vi "False_Predictions.vi"(8 "error in (no error)":errorcluster, 9 "Annotations_for_ClassIdx":T4[](array[typedef]) {"Image Annotations"."BBox"."x" format="%#_4p"; "Image Annotations"."BBox"."y" format="%#_4p"; "Image Annotations"."BBox"."w" format="%#_4p"; "Image Annotations"."BBox"."h" format="%#_4p"}, 10 "TP_IOU_thresh":sgl=0.3, 11 "Detections_for_ClassIdx(by_Image)":T1[](array[typedef]) {"Image Detections"."BBox"."x" format="%#_4p"; "Image Detections"."BBox"."y" format="%#_4p"; "Image Detections"."BBox"."w" format="%#_4p"; "Image Detections"."BBox"."h" format="%#_4p"}) -> (0 "error out":errorcluster, 1 "FPs":cluster{"Array":bool[]}[](array[cluster])=[{"Array"=[FALSE, TRUE]}, {"Array"=[]}, {"Array"=[TRUE]}, {"Array"=[TRUE]}, {"Array"=[FALSE, TRUE, TRUE]}, {"Array"=[FALSE, TRUE, TRUE]}, {"Array"=[]}, {"Array"=[TRUE]}, {"Array"=[TRUE]}, {"Array"=[FALSE]}, {"Array"=[FALSE]}, {"Array"=[FALSE]}, {"Array"=[FALSE]}, {"Array"=[FALSE]}, {"Array"=[TRUE]}, {"Array"=[FALSE]}, {"Array"=[TRUE, TRUE]}, {"Array"=[TRUE, TRUE]}, {"Array"=[FALSE]}, {"Array"=[]}, {"Array"=[FALSE]}, {"Array"=[]}, {"Array"=[]}, {"Array"=[]}, {"Array"=[TRUE]}, {"Array"=[TRUE]}, {"Array"=[TRUE]}, {"Array"=[TRUE]}, {"Array"=[TRUE]}, {"Array"=[]}, {"Array"=[TRUE]}, {"Array"=[TRUE]}, {"Array"=[]}, {"Array"=[]}, {"Array"=[TRUE]}, {"Array"=[TRUE]}, {"Array"=[]}, {"Array"=[]}, {"Array"=[TRUE, FALSE]}, {"Array"=[TRUE, FALSE]}, {"Array"=[TRUE, FALSE, TRUE]}, {"Array"=[]}, {"Array"=[TRUE]}, {"Array"=[TRUE]}, {"Array"=[TRUE]}, {"Array"=[TRUE]}, {"Array"=[TRUE, FALSE]}, {"Array"=[TRUE]}, {"Array"=[TRUE]}, {"Array"=[TRUE]}, {"Array"=[TRUE, FALSE]}, {"Array"=[TRUE]}, {"Array"=[TRUE]}, {"Array"=[TRUE, TRUE]}, {"Array"=[TRUE, TRUE]}, {"Array"=[TRUE, TRUE]}, {"Array"=[TRUE]}, {"Array"=[TRUE, FALSE]}, {"Array"=[TRUE]}, {"Array"=[TRUE, FALSE, TRUE]}, {"Array"=[TRUE, TRUE]}, {"Array"=[TRUE, TRUE]}, {"Array"=[TRUE]}, {"Array"=[TRUE, TRUE]}, {"Array"=[TRUE, TRUE]}, {"Array"=[FALSE, TRUE]}, {"Array"=[TRUE, TRUE]}, {"Array"=[FALSE, TRUE]}, {"Array"=[]}, {"Array"=[]}, {"Array"=[]}, {"Array"=[TRUE]}, {"Array"=[TRUE]}, {"Array"=[]}, {"Array"=[]}, {"Array"=[TRUE, TRUE]}, {"Array"=[TRUE, TRUE, TRUE, FALSE]}, {"Array"=[TRUE, TRUE, TRUE, FALSE]}, {"Array"=[TRUE, TRUE, TRUE, FALSE]}, {"Array"=[TRUE, TRUE, TRUE, FALSE]}, {"Array"=[TRUE, TRUE]}, {"Array"=[TRUE, TRUE]}, {"Array"=[TRUE, TRUE]}, {"Array"=[]}, {"Array"=[]}, {"Array"=[TRUE]}, {"Array"=[TRUE]}, {"Array"=[TRUE]}, {"Array"=[TRUE]}, {"Array"=[TRUE]}, {"Array"=[TRUE, FALSE]}, {"Array"=[TRUE, FALSE]}, {"Array"=[TRUE]}, {"Array"=[FALSE, FALSE]}, {"Array"=[FALSE, FALSE]}, {"Array"=[TRUE, FALSE]}, {"Array"=[]}, {"Array"=[]}, {"Array"=[]}, {"Array"=[TRUE]}, {"Array"=[TRUE]}, {"Array"=[TRUE]}, {"Array"=[TRUE]}, {"Array"=[TRUE]}, {"Array"=[TRUE]}, {"Array"=[TRUE]}, {"Array"=[TRUE]}, {"Array"=[TRUE]}, {"Array"=[TRUE, TRUE]}, {"Array"=[TRUE, TRUE]}, {"Array"=[TRUE, TRUE]}, {"Array"=[TRUE, TRUE]}, {"Array"=[TRUE, TRUE]}, {"Array"=[TRUE, TRUE]}, {"Array"=[FALSE]}, {"Array"=[FALSE]}, {"Array"=[FALSE]}, {"Array"=[]}, {"Array"=[]}, {"Array"=[]}, {"Array"=[]}, {"Array"=[]}, {"Array"=[]}, {"Array"=[FALSE]}, {"Array"=[FALSE]}, {"Array"=[TRUE, FALSE]}, {"Array"=[]}, {"Array"=[]}, {"Array"=[]}, {"Array"=[]}, {"Array"=[]}, {"Array"=[]}, {"Array"=[FALSE]}, {"Array"=[]}, {"Array"=[]}, {"Array"=[FALSE, FALSE]}, {"Array"=[TRUE, FALSE]}, {"Array"=[TRUE, FALSE]}, {"Array"=[TRUE, FALSE]}, {"Array"=[TRUE]}, {"Array"=[TRUE, FALSE, FALSE]}, {"Array"=[]}, {"Array"=[FALSE]}, {"Array"=[FALSE]}, {"Array"=[FALSE]}, {"Array"=[FALSE]}, {"Array"=[FALSE]}, {"Array"=[]}, {"Array"=[]}, {"Array"=[]}, {"Array"=[]}, {"Array"=[]}, {"Array"=[]}, {"Array"=[]}, {"Array"=[]}, {"Array"=[]}, {"Array"=[]}, {"Array"=[]}, {"Array"=[]}, {"Array"=[]}, {"Array"=[]}, {"Array"=[]}, {"Array"=[FALSE]}, {"Array"=[]}, {"Array"=[]}, {"Array"=[]}, {"Array"=[]}, {"Array"=[FALSE]}, {"Array"=[]}, {"Array"=[]}, {"Array"=[FALSE]}, {"Array"=[]}, {"Array"=[]}, {"Array"=[FALSE]}, {"Array"=[TRUE, TRUE]}, {"Array"=[TRUE, TRUE]}, {"Array"=[TRUE, TRUE]}, {"Array"=[TRUE, TRUE]}, {"Array"=[TRUE, TRUE]}, {"Array"=[TRUE, TRUE]}, {"Array"=[]}, {"Array"=[]}, {"Array"=[FALSE]}, {"Array"=[FALSE]}, {"Array"=[]}, {"Array"=[]}, {"Array"=[]}, {"Array"=[FALSE, FALSE, FALSE]}, {"Array"=[FALSE, FALSE]}, {"Array"=[FALSE, FALSE, FALSE]}, {"Array"=[]}, {"Array"=[FALSE]}, {"Array"=[FALSE]}, {"Array"=[TRUE]}, {"Array"=[]}, {"Array"=[TRUE]}, {"Array"=[FALSE, TRUE]}, {"Array"=[TRUE, FALSE, FALSE, TRUE]}, {"Array"=[FALSE, FALSE, FALSE, TRUE]}, {"Array"=[TRUE]}, {"Array"=[TRUE]}, {"Array"=[FALSE, FALSE, TRUE]}, {"Array"=[FALSE, FALSE]}, {"Array"=[]}, {"Array"=[TRUE]}, {"Array"=[TRUE, TRUE, FALSE]}, {"Array"=[TRUE, TRUE, TRUE, TRUE]}, {"Array"=[TRUE, TRUE, FALSE, FALSE]}, {"Array"=[TRUE, TRUE, TRUE, FALSE]}, {"Array"=[TRUE, TRUE]}, {"Array"=[TRUE, TRUE]}, {"Array"=[TRUE, TRUE]}, {"Array"=[TRUE, TRUE]}, {"Array"=[TRUE, TRUE, TRUE]}, {"Array"=[FALSE, TRUE, TRUE]}, {"Array"=[TRUE, TRUE, TRUE, TRUE]}, {"Array"=[TRUE, TRUE, TRUE, TRUE]}, {"Array"=[TRUE, TRUE, TRUE, TRUE]}, {"Array"=[TRUE, TRUE]}, {"Array"=[TRUE, TRUE]}, {"Array"=[TRUE, TRUE, TRUE, TRUE, FALSE]}, {"Array"=[TRUE, TRUE, TRUE, TRUE, FALSE]}, {"Array"=[TRUE, TRUE, TRUE]}, {"Array"=[TRUE, TRUE, TRUE, TRUE, FALSE]}, {"Array"=[TRUE, TRUE, TRUE, FALSE]}, {"Array"=[TRUE, TRUE, TRUE, FALSE]}, {"Array"=[FALSE, TRUE, TRUE]}, {"Array"=[FALSE, TRUE, TRUE, TRUE, FALSE]}, {"Array"=[TRUE, TRUE, FALSE]}, {"Array"=[TRUE, TRUE, FALSE]}, {"Array"=[TRUE, TRUE, FALSE]}, {"Array"=[TRUE, TRUE, FALSE]}, {"Array"=[TRUE, TRUE]}, {"Array"=[TRUE]}, {"Array"=[TRUE, TRUE, TRUE]}, {"Array"=[TRUE, TRUE, TRUE]}, {"Array"=[TRUE, TRUE, TRUE, TRUE]}, {"Array"=[TRUE, TRUE, TRUE]}, {"Array"=[TRUE, TRUE, TRUE]}, {"Array"=[TRUE, TRUE, TRUE]}, {"Array"=[TRUE, TRUE, TRUE]}, {"Array"=[TRUE]}, {"Array"=[TRUE]}, {"Array"=[TRUE]}, {"Array"=[TRUE, TRUE, TRUE]}, {"Array"=[TRUE, TRUE, TRUE]}, {"Array"=[TRUE, TRUE, TRUE]}, {"Array"=[TRUE, TRUE, TRUE]}, {"Array"=[TRUE, TRUE, TRUE]}, {"Array"=[TRUE, TRUE]}, {"Array"=[TRUE, TRUE]}, {"Array"=[TRUE, TRUE]}, {"Array"=[TRUE, TRUE]}, {"Array"=[TRUE, TRUE]}, {"Array"=[TRUE, TRUE]}, {"Array"=[TRUE, TRUE]}, {"Array"=[TRUE, TRUE, TRUE]}, {"Array"=[TRUE, FALSE, TRUE]}, {"Array"=[TRUE, TRUE, TRUE]}, {"Array"=[FALSE, TRUE]}, {"Array"=[TRUE, TRUE]}, {"Array"=[TRUE, TRUE, TRUE]}, {"Array"=[TRUE, TRUE, TRUE]}, {"Array"=[TRUE, TRUE, TRUE]}, {"Array"=[TRUE, TRUE, TRUE]}, {"Array"=[TRUE, TRUE, TRUE, FALSE, TRUE]}, {"Array"=[TRUE, TRUE, TRUE, FALSE]}, {"Array"=[TRUE, TRUE, TRUE, TRUE, FALSE, TRUE]}, {"Array"=[TRUE, TRUE, FALSE, TRUE, TRUE, TRUE]}, {"Array"=[TRUE, TRUE, TRUE, FALSE, TRUE, TRUE]}, {"Array"=[TRUE, TRUE, TRUE, FALSE, TRUE, TRUE]}, {"Array"=[TRUE, TRUE, TRUE, TRUE, FALSE]}, {"Array"=[TRUE]}, {"Array"=[TRUE]}, {"Array"=[TRUE]}, {"Array"=[TRUE, TRUE, FALSE]}, {"Array"=[FALSE, TRUE]}, {"Array"=[TRUE, TRUE, FALSE]}, {"Array"=[TRUE]}, {"Array"=[TRUE]}, {"Array"=[TRUE]}, {"Array"=[TRUE]}, {"Array"=[TRUE]}, {"Array"=[TRUE, FALSE]}, {"Array"=[TRUE, TRUE, FALSE]}, {"Array"=[TRUE, FALSE]}, {"Array"=[TRUE]}, {"Array"=[FALSE, TRUE]}, {"Array"=[TRUE, TRUE, TRUE]}, {"Array"=[TRUE, TRUE]}, {"Array"=[TRUE, TRUE, TRUE, TRUE]}, {"Array"=[TRUE, TRUE, TRUE]}, {"Array"=[TRUE, TRUE, TRUE]}, {"Array"=[TRUE, FALSE, TRUE, TRUE]}, {"Array"=[TRUE, TRUE, TRUE, TRUE, TRUE]}, {"Array"=[TRUE, TRUE, TRUE, TRUE]}, {"Array"=[TRUE, TRUE, TRUE]}, {"Array"=[TRUE, TRUE]}, {"Array"=[TRUE, TRUE, TRUE]}, {"Array"=[TRUE, TRUE, TRUE]}, {"Array"=[TRUE, TRUE]}, {"Array"=[TRUE, TRUE]}, {"Array"=[TRUE, TRUE, FALSE]}, {"Array"=[TRUE, TRUE, FALSE]}, {"Array"=[TRUE, TRUE, TRUE, FALSE]}, {"Array"=[TRUE, TRUE, FALSE]}, {"Array"=[TRUE, FALSE]}, {"Array"=[TRUE, TRUE]}, {"Array"=[TRUE, FALSE]}, {"Array"=[TRUE, FALSE]}, {"Array"=[TRUE, FALSE]}, {"Array"=[TRUE, TRUE]}, {"Array"=[TRUE, TRUE]}, {"Array"=[FALSE, TRUE, TRUE]}, {"Array"=[TRUE, TRUE, TRUE]}, {"Array"=[TRUE, TRUE, TRUE]}, {"Array"=[TRUE, TRUE, TRUE]}, {"Array"=[TRUE, TRUE, FALSE]}, {"Array"=[TRUE, TRUE, TRUE, FALSE]}, {"Array"=[TRUE, FALSE, TRUE]}, {"Array"=[TRUE, FALSE, TRUE]}, {"Array"=[TRUE, FALSE, TRUE]}, {"Array"=[TRUE, TRUE, FALSE]}, {"Array"=[FALSE, TRUE, FALSE, TRUE]}, {"Array"=[TRUE, TRUE]}, {"Array"=[TRUE, FALSE, TRUE]}, {"Array"=[TRUE]}, {"Array"=[TRUE]}, {"Array"=[TRUE, TRUE, TRUE]}, {"Array"=[TRUE, FALSE, TRUE]}, {"Array"=[TRUE, FALSE]}, {"Array"=[TRUE, FALSE, TRUE]}, {"Array"=[TRUE, TRUE, TRUE, TRUE]}, {"Array"=[TRUE, TRUE, TRUE, TRUE]}, {"Array"=[FALSE, TRUE, TRUE, FALSE, TRUE]}, {"Array"=[FALSE, TRUE, TRUE, TRUE, FALSE, TRUE]}, {"Array"=[FALSE, TRUE, TRUE, TRUE]}, {"Array"=[TRUE, FALSE, TRUE, TRUE, TRUE, TRUE]}, {"Array"=[FALSE, TRUE, TRUE]}, {"Array"=[TRUE, TRUE]}, {"Array"=[TRUE, TRUE]}, {"Array"=[TRUE, TRUE, TRUE]}, {"Array"=[TRUE, TRUE, FALSE, TRUE]}, {"Array"=[TRUE, TRUE, TRUE]}, {"Array"=[FALSE, TRUE, TRUE, TRUE]}, {"Array"=[TRUE, FALSE, TRUE, TRUE, TRUE]}, {"Array"=[TRUE, TRUE, TRUE]}, {"Array"=[TRUE, FALSE, TRUE, TRUE]}, {"Array"=[TRUE, TRUE, FALSE]}, {"Array"=[TRUE, TRUE, TRUE]}, {"Array"=[TRUE, TRUE, TRUE, TRUE]}, {"Array"=[TRUE, TRUE, TRUE, TRUE]}, {"Array"=[TRUE, TRUE, TRUE, TRUE]}, {"Array"=[TRUE, TRUE, TRUE, TRUE]}, {"Array"=[TRUE, FALSE, FALSE, TRUE, TRUE]}, {"Array"=[TRUE, FALSE, FALSE, TRUE, TRUE]}, {"Array"=[TRUE, TRUE, TRUE]}, {"Array"=[TRUE, TRUE, FALSE, TRUE]}, {"Array"=[TRUE, TRUE, FALSE, TRUE]}, {"Array"=[TRUE, TRUE, TRUE]}, {"Array"=[TRUE, TRUE, FALSE, TRUE]}, {"Array"=[TRUE, TRUE, FALSE, TRUE]}, {"Array"=[TRUE, TRUE]}, {"Array"=[FALSE, TRUE]}, {"Array"=[FALSE, TRUE]}, {"Array"=[TRUE, FALSE]}, {"Array"=[FALSE, TRUE, TRUE]}, {"Array"=[FALSE, TRUE, TRUE]}, {"Array"=[FALSE, TRUE]}, {"Array"=[TRUE, FALSE, TRUE, TRUE]}, {"Array"=[TRUE, FALSE, TRUE, TRUE]}, {"Array"=[TRUE, TRUE, TRUE, FALSE, TRUE]}, {"Array"=[TRUE, TRUE, TRUE, FALSE, TRUE]}, {"Array"=[TRUE, TRUE, TRUE, FALSE, TRUE, TRUE, TRUE]}, {"Array"=[TRUE, TRUE, TRUE, FALSE, TRUE, FALSE, TRUE]}, {"Array"=[TRUE, TRUE, TRUE, FALSE, TRUE, TRUE, TRUE]}, {"Array"=[FALSE, TRUE, TRUE]}, {"Array"=[FALSE, TRUE, TRUE]}, {"Array"=[FALSE, TRUE, TRUE]}, {"Array"=[TRUE, TRUE, TRUE]}, {"Array"=[FALSE, TRUE, FALSE, TRUE]}, {"Array"=[FALSE, TRUE, FALSE, TRUE]}, {"Array"=[TRUE, TRUE, TRUE, FALSE, TRUE]}, {"Array"=[TRUE, TRUE, TRUE, FALSE, TRUE]}, {"Array"=[TRUE, TRUE, TRUE, TRUE, TRUE, FALSE]}, {"Array"=[TRUE, TRUE, TRUE, TRUE, TRUE, FALSE]}, {"Array"=[TRUE, TRUE, TRUE, TRUE, TRUE, FALSE]}, {"Array"=[TRUE, TRUE, TRUE]}, {"Array"=[TRUE, TRUE, TRUE]}, {"Array"=[TRUE, TRUE, TRUE]}, {"Array"=[TRUE, TRUE, TRUE]}, {"Array"=[TRUE, TRUE, TRUE]}, {"Array"=[TRUE, TRUE, TRUE]}, {"Array"=[TRUE, TRUE, TRUE]}, {"Array"=[TRUE]}, {"Array"=[TRUE, FALSE, FALSE, TRUE]}, {"Array"=[TRUE, FALSE]}, {"Array"=[TRUE, FALSE, TRUE]}, {"Array"=[TRUE, FALSE, TRUE]}, {"Array"=[TRUE, TRUE, TRUE, TRUE]}, {"Array"=[TRUE, TRUE, TRUE]}, {"Array"=[TRUE, FALSE, TRUE]}, {"Array"=[TRUE, FALSE, TRUE, TRUE, TRUE]}, {"Array"=[TRUE, TRUE, TRUE, TRUE, TRUE]}, {"Array"=[TRUE, TRUE, TRUE, TRUE]}, {"Array"=[TRUE, FALSE, TRUE, TRUE, TRUE]}, {"Array"=[TRUE, TRUE, FALSE, TRUE, TRUE, TRUE]}, {"Array"=[TRUE, TRUE, FALSE, TRUE, TRUE, TRUE]}, {"Array"=[TRUE, TRUE, FALSE, TRUE, TRUE, TRUE]}, {"Array"=[TRUE, TRUE, TRUE]}, {"Array"=[FALSE, TRUE, TRUE, TRUE]}, {"Array"=[FALSE, TRUE, TRUE, TRUE]}, {"Array"=[FALSE, TRUE, TRUE, TRUE, TRUE, TRUE]}, {"Array"=[TRUE, TRUE, TRUE, TRUE, TRUE]}, {"Array"=[TRUE, TRUE, TRUE, TRUE, TRUE]}, {"Array"=[TRUE, TRUE, TRUE]}, {"Array"=[TRUE, TRUE, TRUE]}, {"Array"=[TRUE, TRUE, TRUE]}, {"Array"=[TRUE, TRUE, TRUE]}, {"Array"=[TRUE, TRUE, TRUE, TRUE]}, {"Array"=[TRUE, TRUE, TRUE, TRUE]}, {"Array"=[TRUE, TRUE, TRUE, FALSE]}, {"Array"=[TRUE, TRUE, TRUE, TRUE]}, {"Array"=[TRUE, TRUE, TRUE, TRUE]}, {"Array"=[TRUE, TRUE]}, {"Array"=[TRUE, TRUE, TRUE]}, {"Array"=[TRUE, TRUE, TRUE, TRUE]}, {"Array"=[TRUE, TRUE, TRUE, TRUE]}, {"Array"=[TRUE, TRUE, TRUE]}, {"Array"=[TRUE, TRUE, TRUE, TRUE, TRUE]}, {"Array"=[TRUE, TRUE, TRUE, TRUE, FALSE]}, {"Array"=[TRUE, TRUE]}, {"Array"=[TRUE, TRUE]}, {"Array"=[TRUE]}, {"Array"=[TRUE]}, {"Array"=[FALSE]}, {"Array"=[TRUE, TRUE]}, {"Array"=[TRUE, TRUE]}, {"Array"=[TRUE, TRUE]}, {"Array"=[TRUE, TRUE]}, {"Array"=[FALSE, TRUE]}, {"Array"=[TRUE]}, {"Array"=[TRUE, TRUE, TRUE]}, {"Array"=[TRUE, TRUE, TRUE]}, {"Array"=[TRUE, FALSE, TRUE]}, {"Array"=[TRUE, TRUE]}, {"Array"=[TRUE, TRUE]}, {"Array"=[TRUE, FALSE, TRUE, TRUE, FALSE]}, {"Array"=[TRUE, TRUE]}, {"Array"=[TRUE, TRUE, TRUE]}, {"Array"=[TRUE, TRUE, TRUE]}, {"Array"=[TRUE, TRUE]}, {"Array"=[TRUE, TRUE]}, {"Array"=[FALSE, TRUE]}, {"Array"=[TRUE, TRUE]}, {"Array"=[FALSE, TRUE, TRUE]}, {"Array"=[TRUE, TRUE]}], 2 "FNs":cluster{"Array":bool[]}[](array[cluster])=[{"Array"=[FALSE, TRUE]}, {"Array"=[FALSE, FALSE]}, {"Array"=[TRUE, FALSE]}, {"Array"=[TRUE, FALSE]}, {"Array"=[TRUE, FALSE, TRUE]}, {"Array"=[TRUE, FALSE, TRUE]}, {"Array"=[FALSE, FALSE, FALSE]}, {"Array"=[TRUE, FALSE, FALSE]}, {"Array"=[TRUE, FALSE, FALSE]}, {"Array"=[FALSE]}, {"Array"=[FALSE]}, {"Array"=[FALSE]}, {"Array"=[FALSE]}, {"Array"=[FALSE, FALSE]}, {"Array"=[TRUE, FALSE]}, {"Array"=[FALSE, FALSE]}, {"Array"=[TRUE, FALSE, TRUE]}, {"Array"=[TRUE, FALSE, TRUE]}, {"Array"=[FALSE, FALSE, FALSE]}, {"Array"=[FALSE, FALSE, FALSE]}, {"Array"=[FALSE, FALSE, FALSE]}, {"Array"=[FALSE]}, {"Array"=[FALSE]}, {"Array"=[FALSE]}, {"Array"=[TRUE, FALSE]}, {"Array"=[TRUE, FALSE]}, {"Array"=[TRUE, FALSE]}, {"Array"=[FALSE, TRUE]}, {"Array"=[FALSE, TRUE]}, {"Array"=[FALSE, FALSE]}, {"Array"=[TRUE, FALSE, FALSE]}, {"Array"=[TRUE, FALSE, FALSE]}, {"Array"=[FALSE, FALSE, FALSE]}, {"Array"=[FALSE, FALSE, FALSE]}, {"Array"=[TRUE, FALSE, FALSE]}, {"Array"=[FALSE, TRUE]}, {"Array"=[FALSE, FALSE]}, {"Array"=[FALSE, FALSE]}, {"Array"=[FALSE, FALSE, TRUE]}, {"Array"=[TRUE, FALSE, FALSE]}, {"Array"=[TRUE, TRUE, FALSE]}, {"Array"=[FALSE, FALSE, FALSE]}, {"Array"=[TRUE, FALSE, FALSE]}, {"Array"=[TRUE, FALSE, FALSE]}, {"Array"=[TRUE, FALSE]}, {"Array"=[TRUE, FALSE]}, {"Array"=[TRUE, FALSE]}, {"Array"=[TRUE, FALSE]}, {"Array"=[TRUE, FALSE]}, {"Array"=[TRUE, FALSE]}, {"Array"=[TRUE, FALSE, FALSE]}, {"Array"=[TRUE, FALSE, FALSE]}, {"Array"=[TRUE, FALSE, FALSE]}, {"Array"=[FALSE, TRUE, TRUE]}, {"Array"=[FALSE, TRUE, TRUE]}, {"Array"=[FALSE, TRUE, TRUE]}, {"Array"=[FALSE, TRUE]}, {"Array"=[FALSE, TRUE]}, {"Array"=[FALSE, TRUE]}, {"Array"=[TRUE, FALSE, TRUE]}, {"Array"=[TRUE, FALSE, TRUE]}, {"Array"=[TRUE, FALSE, TRUE]}, {"Array"=[FALSE, TRUE, FALSE]}, {"Array"=[TRUE, TRUE, FALSE]}, {"Array"=[TRUE, TRUE, FALSE]}, {"Array"=[FALSE, FALSE, TRUE]}, {"Array"=[TRUE, FALSE, TRUE]}, {"Array"=[FALSE, FALSE, TRUE]}, {"Array"=[FALSE]}, {"Array"=[FALSE]}, {"Array"=[FALSE]}, {"Array"=[TRUE, FALSE]}, {"Array"=[TRUE, FALSE]}, {"Array"=[FALSE, FALSE]}, {"Array"=[FALSE, FALSE]}, {"Array"=[FALSE, TRUE, TRUE]}, {"Array"=[TRUE, TRUE, TRUE]}, {"Array"=[TRUE, TRUE, TRUE]}, {"Array"=[TRUE, TRUE, TRUE]}, {"Array"=[TRUE, TRUE, TRUE]}, {"Array"=[TRUE, TRUE, FALSE]}, {"Array"=[TRUE, TRUE, FALSE]}, {"Array"=[TRUE, TRUE, FALSE]}, {"Array"=[FALSE]}, {"Array"=[FALSE, FALSE]}, {"Array"=[TRUE, FALSE]}, {"Array"=[TRUE, FALSE]}, {"Array"=[FALSE, TRUE, FALSE]}, {"Array"=[FALSE, TRUE, FALSE]}, {"Array"=[FALSE, TRUE, FALSE]}, {"Array"=[FALSE, FALSE, TRUE]}, {"Array"=[FALSE, FALSE, TRUE]}, {"Array"=[FALSE, FALSE, TRUE]}, {"Array"=[FALSE, FALSE, FALSE]}, {"Array"=[FALSE, FALSE, FALSE]}, {"Array"=[FALSE, FALSE, TRUE]}, {"Array"=[FALSE]}, {"Array"=[FALSE]}, {"Array"=[FALSE]}, {"Array"=[FALSE, TRUE]}, {"Array"=[FALSE, TRUE]}, {"Array"=[FALSE, TRUE]}, {"Array"=[TRUE, FALSE]}, {"Array"=[TRUE, FALSE]}, {"Array"=[TRUE, FALSE]}, {"Array"=[TRUE, FALSE]}, {"Array"=[TRUE, FALSE]}, {"Array"=[TRUE, FALSE]}, {"Array"=[TRUE, TRUE, FALSE]}, {"Array"=[TRUE, TRUE, FALSE]}, {"Array"=[TRUE, TRUE, FALSE]}, {"Array"=[TRUE, TRUE, FALSE]}, {"Array"=[TRUE, TRUE, FALSE]}, {"Array"=[TRUE, TRUE, FALSE]}, {"Array"=[FALSE]}, {"Array"=[FALSE]}, {"Array"=[FALSE]}, {"Array"=[FALSE]}, {"Array"=[FALSE]}, {"Array"=[FALSE]}, {"Array"=[FALSE]}, {"Array"=[FALSE]}, {"Array"=[FALSE]}, {"Array"=[FALSE, FALSE]}, {"Array"=[FALSE, FALSE]}, {"Array"=[FALSE, TRUE]}, {"Array"=[FALSE, FALSE]}, {"Array"=[FALSE, FALSE]}, {"Array"=[FALSE, FALSE]}, {"Array"=[FALSE, FALSE]}, {"Array"=[FALSE, FALSE]}, {"Array"=[FALSE, FALSE]}, {"Array"=[FALSE, FALSE]}, {"Array"=[FALSE, FALSE]}, {"Array"=[FALSE, FALSE]}, {"Array"=[FALSE, FALSE, FALSE]}, {"Array"=[FALSE, TRUE, FALSE]}, {"Array"=[FALSE, TRUE, FALSE]}, {"Array"=[TRUE, FALSE, FALSE]}, {"Array"=[TRUE, FALSE, FALSE]}, {"Array"=[TRUE, FALSE, FALSE]}, {"Array"=[FALSE, FALSE, FALSE]}, {"Array"=[FALSE, FALSE, FALSE]}, {"Array"=[FALSE, FALSE, FALSE]}, {"Array"=[FALSE, FALSE, FALSE]}, {"Array"=[FALSE, FALSE, FALSE]}, {"Array"=[FALSE, FALSE, FALSE]}, {"Array"=[FALSE]}, {"Array"=[FALSE]}, {"Array"=[FALSE]}, {"Array"=[FALSE, FALSE]}, {"Array"=[FALSE, FALSE]}, {"Array"=[FALSE, FALSE]}, {"Array"=[FALSE, FALSE]}, {"Array"=[FALSE, FALSE]}, {"Array"=[FALSE, FALSE]}, {"Array"=[FALSE, FALSE, FALSE]}, {"Array"=[FALSE, FALSE, FALSE]}, {"Array"=[FALSE, FALSE, FALSE]}, {"Array"=[FALSE, FALSE, FALSE]}, {"Array"=[FALSE, FALSE, FALSE]}, {"Array"=[FALSE, FALSE, FALSE]}, {"Array"=[FALSE]}, {"Array"=[FALSE]}, {"Array"=[FALSE]}, {"Array"=[FALSE]}, {"Array"=[FALSE]}, {"Array"=[FALSE]}, {"Array"=[FALSE, FALSE]}, {"Array"=[FALSE, FALSE]}, {"Array"=[FALSE, FALSE]}, {"Array"=[FALSE, FALSE]}, {"Array"=[FALSE, FALSE]}, {"Array"=[FALSE, FALSE]}, {"Array"=[TRUE, TRUE, FALSE]}, {"Array"=[TRUE, TRUE, FALSE]}, {"Array"=[TRUE, TRUE, FALSE]}, {"Array"=[TRUE, TRUE, FALSE]}, {"Array"=[TRUE, TRUE, FALSE]}, {"Array"=[TRUE, TRUE, FALSE]}, {"Array"=[FALSE, FALSE, FALSE]}, {"Array"=[FALSE, FALSE, FALSE]}, {"Array"=[FALSE, FALSE, FALSE]}, {"Array"=[FALSE]}, {"Array"=[FALSE]}, {"Array"=[FALSE]}, {"Array"=[FALSE]}, {"Array"=[FALSE, FALSE]}, {"Array"=[FALSE, FALSE]}, {"Array"=[FALSE, FALSE]}, {"Array"=[FALSE, FALSE]}, {"Array"=[FALSE, FALSE]}, {"Array"=[FALSE, FALSE]}, {"Array"=[FALSE, TRUE]}, {"Array"=[FALSE, FALSE]}, {"Array"=[FALSE, TRUE]}, {"Array"=[TRUE, FALSE, FALSE]}, {"Array"=[TRUE, FALSE, TRUE]}, {"Array"=[TRUE, FALSE, FALSE]}, {"Array"=[TRUE, FALSE, FALSE]}, {"Array"=[TRUE, FALSE, FALSE]}, {"Array"=[TRUE, FALSE, FALSE]}, {"Array"=[FALSE, FALSE, FALSE]}, {"Array"=[FALSE, FALSE, FALSE]}, {"Array"=[FALSE, FALSE, TRUE]}, {"Array"=[TRUE, TRUE]}, {"Array"=[TRUE, TRUE, TRUE, FALSE, TRUE]}, {"Array"=[FALSE, TRUE, FALSE, FALSE, TRUE]}, {"Array"=[FALSE, TRUE, TRUE, FALSE, TRUE]}, {"Array"=[TRUE, TRUE, FALSE]}, {"Array"=[TRUE, TRUE, FALSE]}, {"Array"=[TRUE, TRUE, FALSE]}, {"Array"=[FALSE, TRUE, FALSE, TRUE]}, {"Array"=[TRUE, TRUE, FALSE, TRUE]}, {"Array"=[FALSE, TRUE, FALSE, TRUE]}, {"Array"=[TRUE, TRUE, FALSE, TRUE, TRUE]}, {"Array"=[TRUE, TRUE, FALSE, TRUE, TRUE]}, {"Array"=[TRUE, TRUE, FALSE, TRUE, TRUE]}, {"Array"=[TRUE, TRUE, FALSE]}, {"Array"=[TRUE, TRUE, FALSE]}, {"Array"=[TRUE, TRUE, FALSE, TRUE, TRUE]}, {"Array"=[TRUE, TRUE, FALSE, TRUE, TRUE]}, {"Array"=[TRUE, TRUE, FALSE, TRUE, FALSE]}, {"Array"=[TRUE, TRUE, TRUE, FALSE, TRUE]}, {"Array"=[TRUE, FALSE, TRUE, FALSE, TRUE]}, {"Array"=[TRUE, FALSE, TRUE, FALSE, TRUE]}, {"Array"=[TRUE, TRUE, FALSE, FALSE, FALSE, FALSE]}, {"Array"=[TRUE, TRUE, FALSE, FALSE, TRUE, FALSE]}, {"Array"=[TRUE, FALSE, FALSE, FALSE, TRUE, FALSE]}, {"Array"=[FALSE, TRUE, TRUE]}, {"Array"=[FALSE, TRUE, TRUE]}, {"Array"=[FALSE, TRUE, TRUE]}, {"Array"=[FALSE, FALSE, TRUE, TRUE]}, {"Array"=[FALSE, FALSE, FALSE, TRUE]}, {"Array"=[TRUE, FALSE, TRUE, TRUE]}, {"Array"=[TRUE, TRUE, FALSE, TRUE, FALSE, FALSE]}, {"Array"=[TRUE, TRUE, TRUE, TRUE, FALSE, FALSE]}, {"Array"=[TRUE, TRUE, FALSE, TRUE, FALSE, FALSE]}, {"Array"=[TRUE, TRUE, FALSE, TRUE]}, {"Array"=[TRUE, TRUE, FALSE, TRUE]}, {"Array"=[TRUE, TRUE, FALSE, TRUE]}, {"Array"=[FALSE, TRUE]}, {"Array"=[FALSE, TRUE]}, {"Array"=[FALSE, TRUE]}, {"Array"=[TRUE, TRUE, TRUE, FALSE, FALSE]}, {"Array"=[TRUE, TRUE, TRUE, FALSE, FALSE]}, {"Array"=[TRUE, TRUE, TRUE, FALSE, FALSE]}, {"Array"=[FALSE, TRUE, FALSE, TRUE, TRUE, FALSE]}, {"Array"=[FALSE, TRUE, FALSE, TRUE, TRUE, FALSE]}, {"Array"=[FALSE, FALSE, FALSE, TRUE, TRUE, FALSE]}, {"Array"=[TRUE, TRUE, FALSE, FALSE]}, {"Array"=[TRUE, TRUE, FALSE, FALSE]}, {"Array"=[TRUE, TRUE, FALSE, FALSE]}, {"Array"=[FALSE, TRUE, FALSE, TRUE]}, {"Array"=[FALSE, TRUE, FALSE, TRUE]}, {"Array"=[FALSE, TRUE, FALSE, TRUE]}, {"Array"=[FALSE, TRUE, FALSE, TRUE, TRUE]}, {"Array"=[FALSE, TRUE, FALSE, FALSE, TRUE]}, {"Array"=[FALSE, TRUE, FALSE, TRUE, TRUE]}, {"Array"=[FALSE, FALSE, TRUE, FALSE, FALSE]}, {"Array"=[FALSE, FALSE, TRUE, TRUE, FALSE]}, {"Array"=[TRUE, FALSE, TRUE, TRUE, FALSE]}, {"Array"=[TRUE, FALSE, TRUE, TRUE, FALSE, FALSE]}, {"Array"=[FALSE, FALSE, TRUE, TRUE, TRUE, FALSE]}, {"Array"=[TRUE, FALSE, TRUE, TRUE, FALSE, FALSE]}, {"Array"=[TRUE, TRUE, TRUE, TRUE]}, {"Array"=[FALSE, TRUE, TRUE, TRUE]}, {"Array"=[TRUE, TRUE, TRUE, TRUE, TRUE]}, {"Array"=[TRUE, TRUE, TRUE, TRUE, TRUE]}, {"Array"=[TRUE, TRUE, TRUE, FALSE, TRUE, TRUE]}, {"Array"=[TRUE, TRUE, TRUE, FALSE, TRUE, TRUE]}, {"Array"=[FALSE, TRUE, TRUE, FALSE, TRUE, TRUE]}, {"Array"=[FALSE, FALSE, TRUE]}, {"Array"=[FALSE, FALSE, TRUE]}, {"Array"=[FALSE, FALSE, TRUE]}, {"Array"=[TRUE, FALSE, FALSE, TRUE]}, {"Array"=[TRUE, FALSE, FALSE, FALSE]}, {"Array"=[TRUE, TRUE, FALSE, FALSE]}, {"Array"=[FALSE, FALSE, TRUE, FALSE, FALSE]}, {"Array"=[FALSE, FALSE, TRUE, FALSE, FALSE]}, {"Array"=[FALSE, FALSE, TRUE, FALSE, FALSE]}, {"Array"=[TRUE, FALSE, FALSE]}, {"Array"=[TRUE, FALSE, FALSE]}, {"Array"=[TRUE, FALSE, FALSE]}, {"Array"=[TRUE, FALSE, TRUE, FALSE]}, {"Array"=[TRUE, FALSE, FALSE, FALSE]}, {"Array"=[TRUE, FALSE, FALSE, FALSE]}, {"Array"=[FALSE, FALSE, TRUE, FALSE, FALSE, FALSE]}, {"Array"=[TRUE, FALSE, TRUE, TRUE, FALSE, FALSE]}, {"Array"=[TRUE, FALSE, TRUE, FALSE, FALSE, FALSE]}, {"Array"=[TRUE, TRUE, FALSE, TRUE, TRUE]}, {"Array"=[TRUE, TRUE, FALSE, FALSE, TRUE]}, {"Array"=[TRUE, TRUE, FALSE, FALSE, TRUE]}, {"Array"=[TRUE, TRUE, FALSE, FALSE, FALSE, TRUE]}, {"Array"=[TRUE, TRUE, TRUE, FALSE, TRUE, TRUE]}, {"Array"=[TRUE, TRUE, TRUE, FALSE, FALSE, TRUE]}, {"Array"=[FALSE, TRUE, TRUE, TRUE]}, {"Array"=[FALSE, FALSE, TRUE, TRUE]}, {"Array"=[FALSE, TRUE, TRUE, TRUE]}, {"Array"=[TRUE, TRUE, TRUE, FALSE, FALSE]}, {"Array"=[TRUE, FALSE, TRUE, FALSE, FALSE]}, {"Array"=[TRUE, FALSE, TRUE, FALSE, FALSE]}, {"Array"=[FALSE, FALSE, TRUE, FALSE, FALSE, TRUE]}, {"Array"=[FALSE, FALSE, TRUE, FALSE, FALSE, TRUE]}, {"Array"=[FALSE, TRUE, TRUE, FALSE, FALSE, TRUE]}, {"Array"=[TRUE, FALSE, FALSE, FALSE, TRUE]}, {"Array"=[FALSE, FALSE, FALSE, FALSE, TRUE]}, {"Array"=[TRUE, FALSE, FALSE, FALSE, TRUE]}, {"Array"=[FALSE, FALSE, FALSE, FALSE, FALSE, TRUE]}, {"Array"=[FALSE, FALSE, FALSE, FALSE, FALSE, TRUE]}, {"Array"=[FALSE, FALSE, FALSE, FALSE, FALSE, TRUE]}, {"Array"=[TRUE, TRUE, FALSE, FALSE]}, {"Array"=[TRUE, TRUE, FALSE, FALSE]}, {"Array"=[TRUE, TRUE, FALSE, FALSE]}, {"Array"=[FALSE, FALSE, TRUE, TRUE, TRUE]}, {"Array"=[FALSE, FALSE, TRUE, TRUE, TRUE]}, {"Array"=[FALSE, FALSE, TRUE, TRUE, TRUE]}, {"Array"=[TRUE, FALSE, FALSE, TRUE]}, {"Array"=[TRUE, FALSE, TRUE, TRUE]}, {"Array"=[TRUE, FALSE, FALSE, TRUE]}, {"Array"=[TRUE, FALSE, TRUE, FALSE, FALSE, FALSE]}, {"Array"=[TRUE, FALSE, TRUE, FALSE, FALSE, FALSE]}, {"Array"=[TRUE, FALSE, TRUE, FALSE, FALSE, FALSE]}, {"Array"=[TRUE, TRUE, FALSE, FALSE]}, {"Array"=[TRUE, TRUE, FALSE, FALSE]}, {"Array"=[TRUE, TRUE, FALSE, FALSE]}, {"Array"=[TRUE, FALSE, FALSE, FALSE, FALSE]}, {"Array"=[TRUE, FALSE, FALSE, FALSE, FALSE]}, {"Array"=[TRUE, TRUE, FALSE, TRUE, FALSE]}, {"Array"=[FALSE, TRUE, TRUE, FALSE, FALSE, FALSE]}, {"Array"=[FALSE, FALSE, TRUE, FALSE, FALSE, FALSE]}, {"Array"=[FALSE, TRUE, TRUE, FALSE, FALSE, FALSE]}, {"Array"=[FALSE, TRUE, TRUE, TRUE, TRUE]}, {"Array"=[FALSE, TRUE, TRUE, TRUE, TRUE]}, {"Array"=[FALSE, TRUE, FALSE, TRUE, TRUE]}, {"Array"=[TRUE, TRUE, FALSE, FALSE, TRUE, TRUE]}, {"Array"=[TRUE, FALSE, FALSE, FALSE, TRUE, TRUE]}, {"Array"=[TRUE, TRUE, FALSE, TRUE, TRUE, TRUE]}, {"Array"=[TRUE, TRUE, FALSE, FALSE]}, {"Array"=[TRUE, FALSE, FALSE, TRUE]}, {"Array"=[TRUE, TRUE, FALSE, FALSE]}, {"Array"=[FALSE, TRUE, TRUE, TRUE, FALSE]}, {"Array"=[TRUE, TRUE, FALSE, TRUE, FALSE]}, {"Array"=[TRUE, TRUE, FALSE, TRUE, FALSE]}, {"Array"=[FALSE, TRUE, TRUE, TRUE, FALSE, FALSE]}, {"Array"=[TRUE, TRUE, TRUE, TRUE, FALSE, FALSE]}, {"Array"=[TRUE, TRUE, TRUE, FALSE, FALSE, FALSE]}, {"Array"=[TRUE, FALSE, TRUE, TRUE]}, {"Array"=[FALSE, FALSE, TRUE, TRUE]}, {"Array"=[TRUE, FALSE, TRUE, TRUE]}, {"Array"=[TRUE, TRUE, TRUE, TRUE, FALSE]}, {"Array"=[TRUE, TRUE, TRUE, TRUE, FALSE]}, {"Array"=[TRUE, TRUE, TRUE, TRUE, FALSE]}, {"Array"=[FALSE, TRUE, TRUE, TRUE, FALSE, TRUE]}, {"Array"=[FALSE, TRUE, TRUE, FALSE, FALSE, TRUE]}, {"Array"=[FALSE, TRUE, TRUE, FALSE, FALSE, TRUE]}, {"Array"=[TRUE, TRUE, FALSE, TRUE, FALSE]}, {"Array"=[TRUE, TRUE, FALSE, TRUE, FALSE]}, {"Array"=[TRUE, TRUE, FALSE, TRUE, FALSE]}, {"Array"=[TRUE, TRUE, TRUE, FALSE, FALSE, FALSE]}, {"Array"=[TRUE, TRUE, TRUE, FALSE, FALSE, FALSE]}, {"Array"=[TRUE, TRUE, TRUE, FALSE, FALSE, FALSE]}, {"Array"=[TRUE, FALSE, FALSE, TRUE]}, {"Array"=[TRUE, FALSE, FALSE, FALSE]}, {"Array"=[TRUE, FALSE, FALSE, FALSE]}, {"Array"=[FALSE, TRUE, FALSE, FALSE, FALSE]}, {"Array"=[FALSE, FALSE, FALSE, TRUE, TRUE]}, {"Array"=[FALSE, FALSE, FALSE, TRUE, TRUE]}, {"Array"=[TRUE, FALSE, FALSE, FALSE, FALSE, FALSE]}, {"Array"=[TRUE, TRUE, FALSE, TRUE, FALSE, FALSE]}, {"Array"=[TRUE, TRUE, FALSE, TRUE, FALSE, FALSE]}, {"Array"=[TRUE, TRUE, TRUE, FALSE, TRUE]}, {"Array"=[TRUE, TRUE, TRUE, FALSE, TRUE]}, {"Array"=[TRUE, TRUE, TRUE, TRUE, TRUE, TRUE]}, {"Array"=[TRUE, FALSE, TRUE, TRUE, TRUE, TRUE]}, {"Array"=[TRUE, TRUE, TRUE, TRUE, TRUE, TRUE]}, {"Array"=[TRUE, FALSE, FALSE, TRUE]}, {"Array"=[TRUE, FALSE, FALSE, TRUE]}, {"Array"=[TRUE, FALSE, FALSE, TRUE]}, {"Array"=[TRUE, TRUE, FALSE, FALSE, TRUE, FALSE]}, {"Array"=[TRUE, TRUE, FALSE, FALSE, FALSE, FALSE]}, {"Array"=[TRUE, TRUE, FALSE, FALSE, FALSE, FALSE]}, {"Array"=[TRUE, TRUE, FALSE, TRUE, TRUE]}, {"Array"=[TRUE, TRUE, FALSE, TRUE, TRUE]}, {"Array"=[TRUE, TRUE, TRUE, TRUE, TRUE, FALSE]}, {"Array"=[TRUE, TRUE, TRUE, TRUE, TRUE, FALSE]}, {"Array"=[TRUE, TRUE, TRUE, TRUE, TRUE, FALSE]}, {"Array"=[TRUE, TRUE, TRUE, FALSE]}, {"Array"=[TRUE, TRUE, TRUE, FALSE]}, {"Array"=[TRUE, TRUE, TRUE, FALSE]}, {"Array"=[TRUE, FALSE, TRUE, TRUE, FALSE]}, {"Array"=[TRUE, TRUE, FALSE, TRUE, FALSE]}, {"Array"=[TRUE, TRUE, FALSE, TRUE, FALSE]}, {"Array"=[FALSE, FALSE, TRUE, TRUE, TRUE, FALSE]}, {"Array"=[FALSE, FALSE, FALSE, FALSE, TRUE, FALSE]}, {"Array"=[FALSE, FALSE, TRUE, FALSE, TRUE, FALSE]}, {"Array"=[TRUE, FALSE, FALSE, FALSE]}, {"Array"=[TRUE, FALSE, TRUE, FALSE]}, {"Array"=[TRUE, FALSE, TRUE, FALSE]}, {"Array"=[FALSE, TRUE, TRUE, TRUE, TRUE]}, {"Array"=[FALSE, FALSE, TRUE, TRUE, TRUE]}, {"Array"=[FALSE, FALSE, TRUE, FALSE, TRUE]}, {"Array"=[TRUE, TRUE, TRUE, FALSE, FALSE, TRUE]}, {"Array"=[TRUE, TRUE, TRUE, TRUE, FALSE, TRUE]}, {"Array"=[TRUE, FALSE, TRUE, TRUE, FALSE, TRUE]}, {"Array"=[TRUE, TRUE, FALSE, TRUE, TRUE]}, {"Array"=[TRUE, TRUE, TRUE, TRUE, FALSE, TRUE]}, {"Array"=[TRUE, TRUE, TRUE, TRUE, FALSE, TRUE]}, {"Array"=[TRUE, TRUE, TRUE, TRUE, FALSE, TRUE]}, {"Array"=[TRUE, FALSE, TRUE, TRUE]}, {"Array"=[TRUE, FALSE, TRUE, TRUE]}, {"Array"=[TRUE, FALSE, TRUE, TRUE]}, {"Array"=[TRUE, TRUE, TRUE, TRUE, TRUE, FALSE]}, {"Array"=[TRUE, TRUE, TRUE, TRUE, TRUE, FALSE]}, {"Array"=[TRUE, TRUE, TRUE, TRUE, TRUE, FALSE]}, {"Array"=[TRUE, TRUE, TRUE, FALSE]}, {"Array"=[TRUE, TRUE, TRUE, FALSE]}, {"Array"=[TRUE, TRUE, TRUE, FALSE]}, {"Array"=[TRUE, TRUE, FALSE, FALSE, TRUE]}, {"Array"=[TRUE, TRUE, TRUE, FALSE, TRUE]}, {"Array"=[TRUE, TRUE, TRUE, FALSE, TRUE]}, {"Array"=[FALSE, TRUE, TRUE, FALSE, TRUE, FALSE]}, {"Array"=[TRUE, TRUE, TRUE, FALSE, TRUE, FALSE]}, {"Array"=[TRUE, TRUE, TRUE, FALSE, TRUE, FALSE]}, {"Array"=[TRUE, TRUE, FALSE, FALSE]}, {"Array"=[TRUE, TRUE, TRUE, FALSE]}, {"Array"=[TRUE, TRUE, TRUE, FALSE, TRUE]}, {"Array"=[TRUE, TRUE, TRUE, FALSE, TRUE]}, {"Array"=[TRUE, TRUE, FALSE, FALSE, TRUE]}, {"Array"=[FALSE, TRUE, TRUE, TRUE, TRUE, TRUE]}, {"Array"=[FALSE, TRUE, FALSE, TRUE, TRUE, TRUE]}, {"Array"=[FALSE, TRUE, TRUE]}, {"Array"=[FALSE, TRUE, TRUE]}, {"Array"=[FALSE, TRUE, FALSE, FALSE]}, {"Array"=[FALSE, TRUE, FALSE, FALSE]}, {"Array"=[FALSE, FALSE, FALSE, FALSE]}, {"Array"=[FALSE, FALSE, TRUE, FALSE, TRUE]}, {"Array"=[FALSE, FALSE, TRUE, FALSE, TRUE]}, {"Array"=[FALSE, FALSE, TRUE, FALSE, TRUE]}, {"Array"=[FALSE, TRUE, FALSE, FALSE, FALSE, TRUE]}, {"Array"=[FALSE, FALSE, FALSE, FALSE, FALSE, TRUE]}, {"Array"=[FALSE, FALSE, FALSE, FALSE, FALSE, TRUE]}, {"Array"=[TRUE, FALSE, TRUE, TRUE, FALSE]}, {"Array"=[TRUE, FALSE, TRUE, TRUE, FALSE]}, {"Array"=[TRUE, FALSE, FALSE, TRUE, FALSE]}, {"Array"=[FALSE, TRUE, FALSE, FALSE, FALSE, TRUE]}, {"Array"=[FALSE, TRUE, TRUE, FALSE, FALSE, FALSE]}, {"Array"=[FALSE, TRUE, TRUE, FALSE, FALSE, TRUE]}, {"Array"=[FALSE, TRUE, FALSE, TRUE, FALSE, FALSE]}, {"Array"=[TRUE, TRUE, FALSE, TRUE, FALSE, FALSE]}, {"Array"=[TRUE, TRUE, FALSE, TRUE, FALSE, FALSE]}, {"Array"=[TRUE, TRUE, FALSE, FALSE, FALSE]}, {"Array"=[TRUE, TRUE, FALSE, FALSE, FALSE]}, {"Array"=[TRUE, FALSE, FALSE, FALSE, FALSE]}, {"Array"=[TRUE, TRUE, FALSE, FALSE, FALSE, FALSE]}, {"Array"=[TRUE, TRUE, FALSE, FALSE, FALSE, FALSE]}, {"Array"=[TRUE, TRUE, FALSE, FALSE, FALSE, FALSE]}], 3 "Incorrect classified samples":i32[](array[numeric])=[3, 6, 7, 8, 9, 10, 12, 13, 14, 18, 20, 22, 23, 27, 28, 29, 31, 32, 33, 34, 35, 39, 40, 41, 45, 46, 47, 48, 49, 50, 52, 53, 54, 55, 56, 69, 70, 71, 73, 75, 76, 78, 79, 80, 90, 91, 92, 93, 94, 95, 102, 103, 104, 105, 106, 107, 114, 115, 116, 120, 121, 122, 123, 124, 125, 126, 127, 128, 129, 130, 131, 141, 142, 144, 145, 147, 149, 150, 152, 155, 156, 157, 158, 161, 165, 166, 167, 168, 169, 170, 171, 172, 173, 174, 175, 176, 177, 178, 179, 183, 184, 185, 186, 187, 188, 189, 190, 191, 192, 193, 194, 195, 196, 197, 198, 199, 200, 201, 202, 203, 204, 205, 206, 207, 208, 209, 210, 211, 212, 213, 214, 215, 216, 217, 218, 219, 220, 221, 222, 223, 224, 225, 226, 227, 228, 229, 230, 234, 235, 236, 240, 241, 242, 243, 244, 245, 249, 250, 251, 252, 253, 254, 261, 262, 263, 264, 265, 266, 270, 271, 272, 273, 274, 275, 276, 277, 278, 279, 280, 281, 282, 283, 284, 286, 288, 289, 290, 291, 292, 293, 294, 295, 296, 297, 298, 299, 300, 301, 302, 303, 304, 305, 306, 307, 308, 323, 327, 328, 329, 330, 331, 332, 333, 334, 335, 336, 337, 338, 340, 341, 342, 343, 344, 345, 346, 347, 348, 349, 350, 351, 352, 353, 354, 355, 356, 357, 358, 359, 360, 361, 362, 363, 364, 365, 366, 367, 368, 369, 370, 371, 372, 373, 374, 375, 376, 377, 378, 379, 380, 381, 382, 383, 384, 385, 386, 388, 389, 390, 391, 393, 394, 395, 396, 397, 398, 399, 400, 401, 402, 403, 404, 405, 406, 407, 408, 409, 410, 411, 412, 413, 414, 415, 416, 417, 418, 419, 420, 421, 422, 423, 424, 425, 426, 427, 428, 429, 430, 431, 432, 433, 434, 435, 436, 437, 438, 439, 440, 441, 442, 443, 444, 445, 446, 447, 448, 449, 450, 451, 452, 453, 454, 455, 456, 457, 458, 459, 460, 461, 462, 463, 464, 465, 466, 467, 468, 469, 470, 471, 472, 473, 474, 475, 476, 477, 478, 479, 480, 481, 482, 483, 484, 485, 486, 487, 488, 489, 490, 491, 492, 493, 494, 498, 499, 501, 502, 503, 504, 505, 506, 507, 508, 509, 511, 512, 513, 514, 515, 516, 517, 518, 519, 520, 521, 522, 523, 524, 525, 526, 527, 528, 529, 530, 531, 532, 533, 536, 537, 538, 539, 546, 547, 548, 549, 550, 551, 552, 553, 554, 555, 556, 557, 558, 559, 560, 561, 563, 564, 565, 566, 567, 569, 573, 575, 576, 577, 578, 579, 580, 581, 582, 583, 584, 585, 586, 587, 588, 589, 590, 591, 592, 593, 594, 595, 596, 597, 598, 599], 4 "#FP":i32=354, 5 "Recall":dbl=0.7762762762762763, 6 "#FN":i32=447, 7 "Precision":dbl=0.7299771167048055)   [LabVIEW 2020]
uses:
  <vilib>/Ngene/Deep Learning Toolkit/Toolkit/NN_Data/API/Data/Detection_Types/NN_Image_Annotations.ctl
  <vilib>/Ngene/Deep Learning Toolkit/Toolkit/NN_Data/API/Data/Detection_Types/NN_BBox_Annotation.ctl
  <vilib>/Ngene/Deep Learning Toolkit/Toolkit/NN_Data/API/Data/Detection_Types/NN_BBox.ctl
  <vilib>/Ngene/Deep Learning Toolkit/Toolkit/NN_Data/API/Data/Detection_Types/NN_Image_Detections.ctl
  <vilib>/Ngene/Deep Learning Toolkit/Toolkit/NN_Data/API/Data/Detection_Types/NN_BBox_Detection.ctl
  <vilib>/Ngene/Deep Learning Toolkit/Toolkit/NN_Layers/Layers/YOLO_v2/SubVIs/NN_BBox_IOU.vi
  <vilib>/Ngene/Deep Learning Toolkit/Toolkit/Deep_Learning_Toolkit_by_Ngene.lvlib
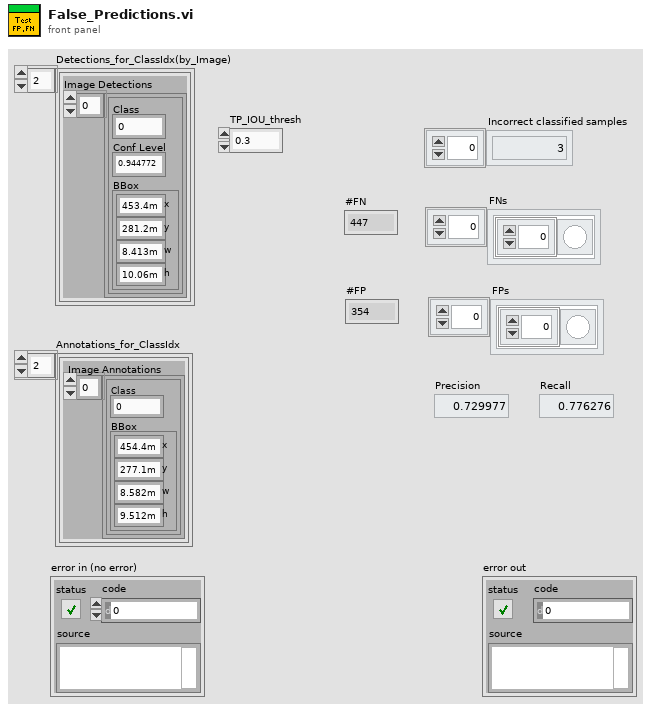
[diagram p1: front panel]
types:
  T1 = typedef "Deep_Learning_Toolkit_by_Ngene.lvlib/NN_Image_Detections.ctl" = cluster{"Image Detections":T2[]}
  T2 = typedef "Deep_Learning_Toolkit_by_Ngene.lvlib/NN_BBox_Detection.ctl" = cluster{"Class":i32, "Conf Level":sgl, "BBox":T3}
  T3 = typedef "Deep_Learning_Toolkit_by_Ngene.lvlib/NN_BBox.ctl" = cluster{"x":sgl, "y":sgl, "w":sgl, "h":sgl}
  T4 = typedef "Deep_Learning_Toolkit_by_Ngene.lvlib/NN_Image_Annotations.ctl" = cluster{"Image Annotations":T5[]}
  T5 = typedef "Deep_Learning_Toolkit_by_Ngene.lvlib/NN_BBox_Annotation.ctl" = cluster{"Class":i32, "BBox":T3}
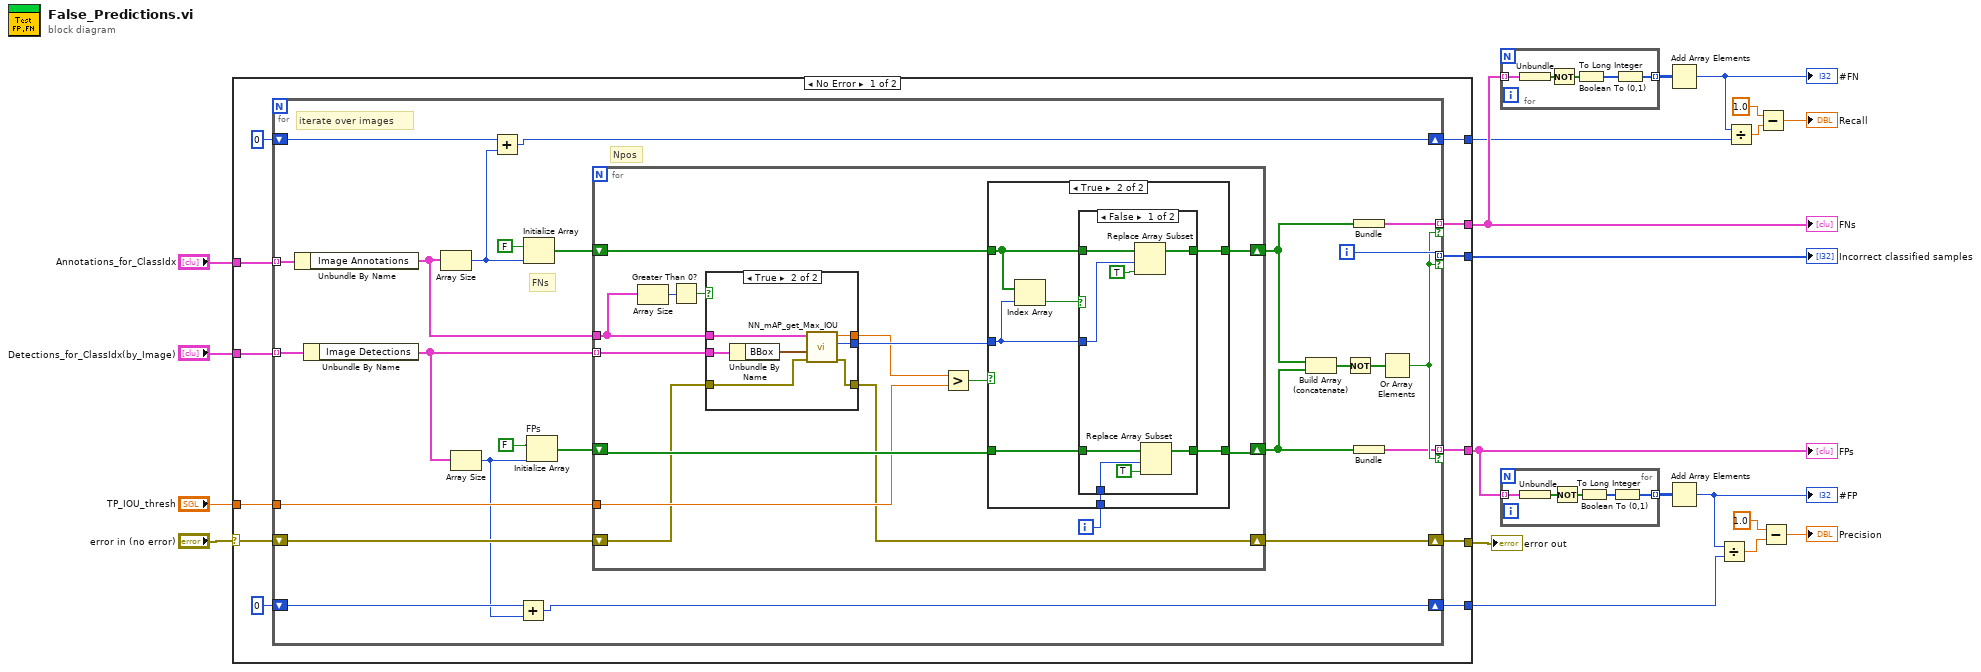
[diagram p0: block diagram]
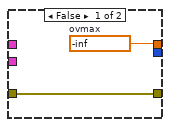
[diagram p4: hidden frame]
diagram:
  n1 = case shown="No Error" "error in (no error)" {
    selector: "error in (no error)" -> [w32 w101]
    tunnel: "TP_IOU_thresh" -> [w21 _]
    tunnel: "Detections_for_ClassIdx(by_Image)" -> [w29 _]
    tunnel: "Annotations_for_ClassIdx" -> [w30 _]
    tunnel: [w31 w101] -> w18
    tunnel: [w28 _] -> w17
    tunnel: [w27 _] -> w9
    tunnel: [w26 _] -> w4
    tunnel: [w24 _] -> w2
    tunnel: [w22 _] -> w1
    frame No Error {
      n2 = for {
        tunnel: w30 -> [w54] mode=indexing
        tunnel: w21 -> [w53]
        tunnel: w29 -> [w52] mode=indexing
        shift-right: [w55] -> w31
        shift-left: w32 -> [w56]
        tunnel: [w46] -> w28 mode=indexing if=w41
        tunnel: [w40] -> w27 mode=indexing if=w41
        tunnel: [w39] -> w26 mode=indexing if=w41
        shift-right: [w36] -> w24
        shift-left: 0 -> [w37]
        shift-right: [w33] -> w22
        shift-left: 0 -> [w35]
        i -> [w46]
        # "FNs"
        # "iterate over images"
        # "Npos"
        n3 = Unbundle By Name(w54) -> ("Image Annotations"=w49:T5[])
        n4 = Unbundle By Name(w52) -> ("Image Detections"=w50:T2[])
        n5 = Array Size(array=w49) -> (size(s)=w38:i32)
        n6 = Array Size(array=w50) -> (size(s)=w34:i32)
        n7 = Add(x=w37, y=w38) -> (x+y=w36:i32)
        n8 = Add(x=w35, y=w34) -> (x+y=w33:i32)
        n9 = Initialize Array(FALSE, w38) -> (w48:bool[])
        n10 = Initialize Array "FPs"(FALSE, w34) -> (w57:bool[])
        n11 = for {
          tunnel: w53 -> [w68]
          shift-right: [w72] -> w42
          shift-left: w57 -> [w71]
          tunnel: w50 -> [w64] mode=indexing
          shift-right: [w62] -> w55
          shift-left: w56 -> [w63]
          tunnel: w49 -> [w61]
          shift-right: [w59] -> w43
          shift-left: w48 -> [w60]
          i -> [w58]
          n12 = Array Size(array=w61) -> (size(s)=w66:i32)
          n13 = Greater Than 0?(x=w66) -> (x > 0?=w65:bool)
          n14 = case shown="True" w65 {
            tunnel: [w93 w99] -> w67
            tunnel: [_ w100] -> w69
            tunnel: w61 -> [_ w98]
            tunnel: w64 -> [_ w96]
            tunnel: w63 -> [w92 w95]
            tunnel: [w92 w94] -> w62
            frame False {
              w93 = sgl -inf  # ovmax
            }
            frame True {
              n15 = Unbundle By Name(w96) -> ("BBox"=w97:T3)
              n16 = call <vilib>:"NN_mAP_get_Max_IOU.vi"("error in (no error)"=w95, "Detection Box"=w97, "Annotations"=w98) -> ("error out"=w94:errorcluster, "Max_Index"=w100:i32, "Max_IOU"=w99:sgl)  [unwired: 6 in]
            }
          }
          n17 = Greater?(x=w67, y=w68) -> (0:w70:bool)
          n18 = case shown="True" w70 {
            tunnel: w71 -> [w74 w81]
            tunnel: [w74 w80] -> w72
            tunnel: w69 -> [_ w79]
            tunnel: w60 -> [w73 w78]
            tunnel: [w73 w77] -> w59
            tunnel: w58 -> [_ w76]
            frame False {
            }
            frame True {
              n19 = Index Array(array=w78, index=w79) -> (element=w75:bool)
              n20 = case shown="False" w75 {
                tunnel: w81 -> [w85 w91]
                tunnel: [w84 w91] -> w80
                tunnel: w79 -> [w88 _]
                tunnel: [w86 w90] -> w77
                tunnel: w78 -> [w87 w90]
                tunnel: w76 -> [w83 _]
                frame False {
                  n21 = Replace Array Subset(array=w87, new element=TRUE ("new element/subarray"), index=w88) -> (w86:bool[])
                  n22 = Replace Array Subset(array=w85, new element=TRUE ("new element/subarray"), index=w83) -> (w84:bool[])
                }
                frame True {
                }
              }
            }
          }
        }
        n23 = Build Array (concatenate)(w43, w42) -> (w45:bool[])
        n24 = Not(x=w45) -> (.not. x?=w44:bool[])
        n25 = Bundle(w43) -> (w40:cluster{bool[]})  [unwired: 1 in]
        n26 = Bundle(w42) -> (w39:cluster{bool[]})  [unwired: 1 in]
        n27 = Or Array Elements(Boolean array=w44) -> (logical OR=w41:bool)
      }
    }
    frame Error {
    }
  }
  "error out" <- w18
  "Incorrect classified samples" <- w17
  "FNs" <- w9
  "FPs" <- w4
  n28 = for {
    tunnel: w9 -> [w106] mode=indexing
    tunnel: [w103] -> w10 mode=indexing
    n29 = Unbundle(w106) -> (w105:bool[])
    n30 = Not(x=w105) -> (.not. x?=w102:bool[])
    n31 = Boolean To (0,1)(Boolean=w102) -> (0, 1=w104:i16[])
    n32 = To Long Integer(number=w104) -> (32bit integer=w103:i32[])
  }
  n33 = for {
    tunnel: w4 -> [w111] mode=indexing
    tunnel: [w109] -> w5 mode=indexing
    n34 = Unbundle(w111) -> (w110:bool[])
    n35 = Not(x=w110) -> (.not. x?=w108:bool[])
    n36 = Boolean To (0,1)(Boolean=w108) -> (0, 1=w107:i16[])
    n37 = To Long Integer(number=w107) -> (32bit integer=w109:i32[])
  }
  n38 = Add Array Elements(numeric array=w10) -> (sum=w7:i32)
  "#FN" <- w7
  n39 = Add Array Elements(numeric array=w5) -> (sum=w3:i32)
  "#FP" <- w3
  n40 = Divide(x=w3, y=w1) -> (x/y=w15:dbl)
  n41 = Divide(x=w7, y=w2) -> (x/y=w12:dbl)
  n42 = Subtract(x=1.0, y=w12) -> (x-y=→"Recall":dbl)
  n43 = Subtract(x=1.0, y=w15) -> (x-y=→"Precision":dbl)
